vi "Create Alarm From Code And Add To Active Alarms.vi"(8 "error in (no error)":errorcluster, 10 "Numeric":i32, 11 "Alarm Handler Actor in":refnum<class "Alarm Handler Actor.lvclass">) -> (0 "error out":errorcluster, 3 "Alarm Handler Actor out":refnum<class "Alarm Handler Actor.lvclass">)   [LabVIEW 2015, in "Alarm Handler Actor.lvclass"]
uses:
  Alarm Handler Actor.lvclass
  Active Alarm.ctl
  Alarm Details.ctl
  Alarm Handler Actor.lvclass/Alarm Handler Actor.ctl
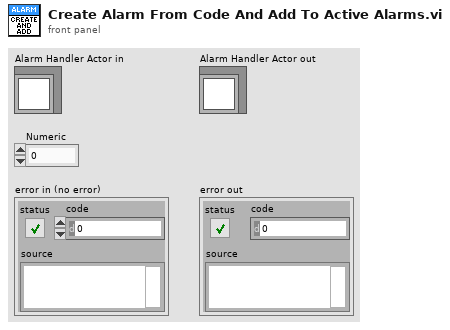
[diagram p1: front panel]
types:
  T1 = typedef "Alarm Handler Actor.lvclass/Active Alarm.ctl" = cluster{"Alarm Detail":T2, "Count":i32, "First Error":timestamp, "Last Error":timestamp, "LabVIEW Error":bool}
  T2 = typedef "Alarm Handler Actor.lvclass/Alarm Details.ctl" = cluster{"Code":i32, "Loop":i32, "Description":string, "Severity":i32, "Clear on Ack?":bool, "Log All Events?":bool}
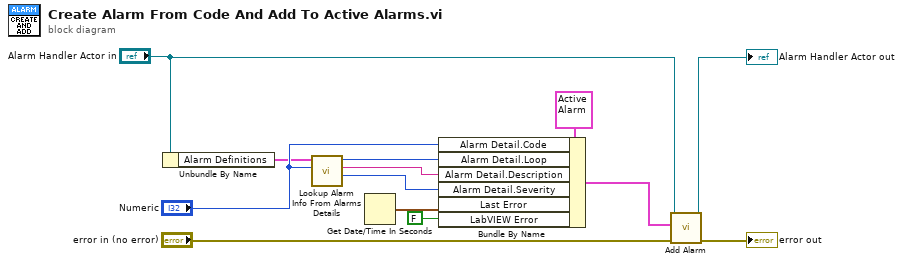
[diagram p0: block diagram]
diagram:
  n1 = Unbundle By Name("Alarm Handler Actor in") -> ("Alarm Definitions"=w1:T2[])
  n2 = call "Lookup Alarm Info From Alarms Details.vi"("Code"="Numeric", "Alarm Details"=w1) -> ("Severity"=w7:i32, "Description"=w6:string, "Loop"=w5:i32)  [unwired: 7 in]
  n3 = Get Date/Time In Seconds() -> (seconds since 1Jan1904=w3:timestamp)
  n4 = Bundle By Name(cluster=T1 {"Alarm Detail"={"Code"=0, "Loop"=0, "Description"="", "Severity"=0, "Clear on Ack?"=FALSE, "Log All Events?"=FALSE}, "Count"=0, "First Error"=timestamp(0 s since 1904-01-01), "Last Error"=timestamp(0 s since 1904-01-01), "LabVIEW Error"=FALSE} ("Present Alarm"), "Alarm Detail.Code"="Numeric", "Alarm Detail.Loop"=w5, "Alarm Detail.Description"=w6, "Alarm Detail.Severity"=w7, "Last Error"=w3, "LabVIEW Error"=FALSE ("LV error")) -> (w11:T1)
  n5 = call "Add Alarm.vi"("error in (no error)"="error in (no error)", "Alarm"=w11, "Actor in"="Alarm Handler Actor in") -> ("error out"=→"error out":errorcluster, "Actor out"=→"Alarm Handler Actor out":refnum<class "Alarm Handler Actor.lvclass">)  [unwired: 7 in]
